vi "SetRF.vi"(0 "reference in":refnum<class "sim_MmW.lvclass">, 5 "Port":string(combo), 7 "Frequency":dbl format="%#_6pHz", 9 "Gain":dbl format="%#_6fdb", 11 "error in (no error)":errorcluster) -> (4 "reference out":refnum<class "sim_MmW.lvclass">, 15 "error out":errorcluster)   [LabVIEW 2019, in "sim_MmW.lvclass"]
doc: "Set RF configuration for port:\nGain and frequency"
uses:
  sim_MmW.lvclass
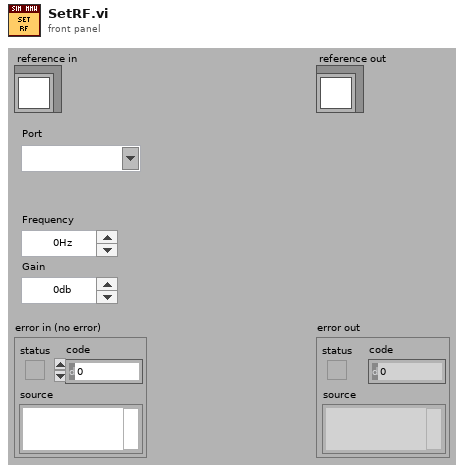
[diagram p1: front panel]
types:
  T1 = typedef "sim_MmW.lvclass/ObjectAttributesRef.ctl" = refnum<data-value>
  T2 = typedef "sim_MmW.lvclass/ObjectAttributes.ctl" = cluster{"RF config":T3, "RX samples":i32, "Downloaded Bursts":map{string, refnum<class "mmWave data.lvclass">}, "TX Fs":dbl, "RX Fs":dbl, "burst sequence":string[], "Burst mode":T4}
  T3 = typedef "mmWave HW Control.lvlib/HW TXRX RF config cluster.ctl" = cluster{"TX.Frequency":dbl, "TX.Gain":dbl, "TX.mmWave adapter":string, "RX.Frequency":dbl, "RX.Gain":dbl, "RX.mmWave adapter":string}
  T4 = typedef "mmWave instrument.lvclass/BurstMode.ctl" = enum16{"burst", "continuous"}
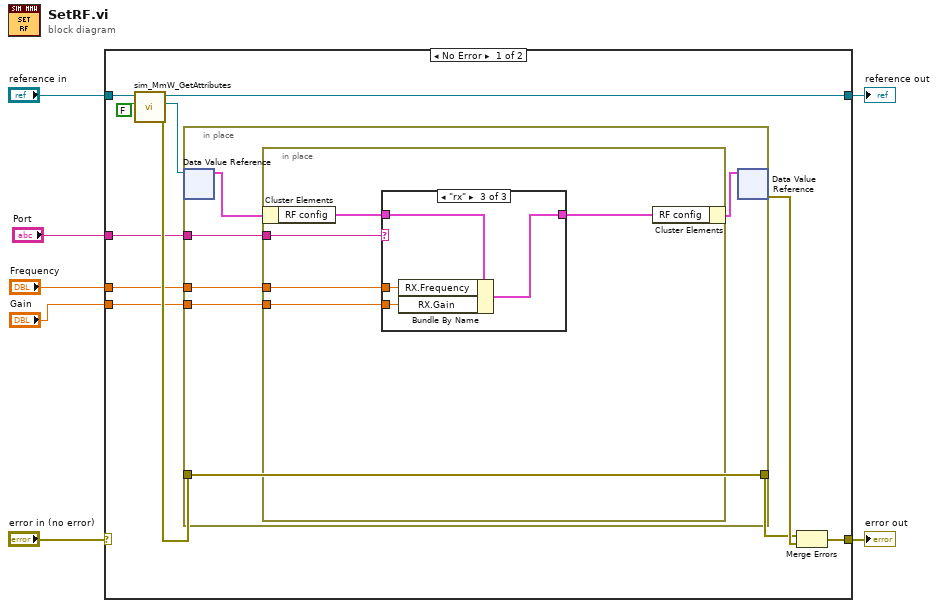
[diagram p0: block diagram]
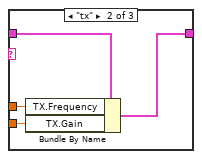
[diagram p3: hidden frame]
diagram:
  n1 = case shown="No Error" "error in (no error)" {
    selector: "error in (no error)" -> [_ w40]
    tunnel: [w18 w40] -> w6
    tunnel: [w12 w39] -> w4
    tunnel: "reference in" -> [w15 w39]
    tunnel: "Port" -> [w10 _]
    tunnel: "Frequency" -> [w9 _]
    tunnel: "Gain" -> [w8 _]
    frame No Error {
      n2 = call "sim_MmW_GetAttributes.vi"("return data? (T)"=FALSE, "reference in"=w15) -> ("error out"=w13:errorcluster, "attributes ref"=w11:T1, "reference out"=w12:refnum<class "sim_MmW.lvclass">)  [unwired: 6 in, 1 out]
      n3 = in-place {
        in-place-border: w13 -> [w22]
        in-place-border: [w22] -> w16
        in-place-border: w10 -> [w21]
        in-place-border: w9 -> [w20]
        in-place-border: w8 -> [w19]
        n4 = in-place-dvr #1(w11) -> (w23:T2)  [unwired: 1 out]
        n5 = in-place {
          in-place-border: w21 -> [w27]
          in-place-border: w20 -> [w26]
          in-place-border: w19 -> [w25]
          n6 = in-place-cluster #2(w23) -> ("RF config"=w28:T3)
          n7 = case shown="\"rx\"" w27 {
            tunnel: [w30 w33 w37] -> w29
            tunnel: w28 -> [w30 w34 w38]
            tunnel: w26 -> [_ w32 w36]
            tunnel: w25 -> [_ w31 w35]
            frame "False", Default {
            }
            frame "tx" {
              n8 = Bundle By Name(cluster=w34, "TX.Frequency"=w32, "TX.Gain"=w31) -> (w33:T3)
            }
            frame "rx" {
              n9 = Bundle By Name(cluster=w38, "RX.Frequency"=w36, "RX.Gain"=w35) -> (w37:T3)
            }
          }
          n10 = in-place-cluster #2("RF config"=w29) -> (w24:T2)
        }
        n11 = in-place-dvr #1(w24) -> (w17:errorcluster)  [unwired: 1 out]
      }
      n12 = Merge Errors(w16, w17) -> (w18:errorcluster)
    }
    frame Error {
    }
  }
  "error out" <- w6
  "reference out" <- w4
